vi "Example.vi"   [LabVIEW 2016, in "Global_logger.lvlib"]
uses:
  Global_logger.lvlib
  Levels.ctl
  Options.ctl
types:
  T1 = typedef "Global_logger.lvlib/Options.ctl" = cluster{"filesize (bytes)":u32, "logs max age (days) ":u16, "write per N messages":u16}
  T2 = typedef "Global_logger.lvlib/Levels.ctl" = enum16{"ALL", "TRACE", "DEBUG", "INFO", "WARN", "ERROR", "FATAL", "OFF"}
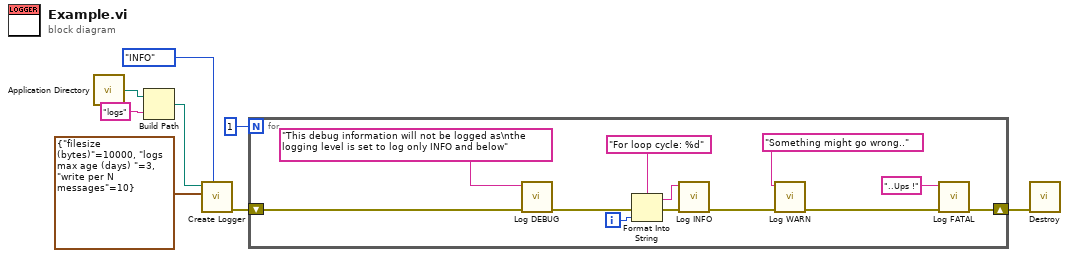
[diagram p0: block diagram]
diagram:
  n1 = call <vilib>:"Application Directory.vi"() -> ("Application Directory"=w6:path)
  n2 = Build Path(base path=w6, name or relative path="logs") -> (appended path=w4:path)
  n3 = call "Create Logger.vi"("Level"=Levels."INFO", "Options"=T1 {"filesize (bytes)"=10000, "logs max age (days) "=3, "write per N messages"=10}, "Root Logging Path"=w4) -> ("error out"=w3:errorcluster)  [unwired: 8 in]
  n4 = for {
    N: 1 -> [_]
    shift-right: [w17] -> w2
    shift-left: w3 -> [w20]
    i -> [w13]
    n5 = call "Log DEBUG.vi"("error in (no error)"=w20, "Message"="This debug information will not be logged as\nthe logging level is set to log only INFO and below") -> ("error out"=w19:errorcluster)  [unwired: 9 in]
    n6 = Format Into String(format string="For loop cycle: %d", error in=w19, w13) -> (resulting string=w11:string, error out=w14:errorcluster)  [unwired: 1 in]
    n7 = call "Log INFO.vi"("error in (no error)"=w14, "Message"=w11) -> ("error out"=w18:errorcluster)  [unwired: 9 in]
    n8 = call "Log WARN.vi"("error in (no error)"=w18, "Message"="Something might go wrong.." ("format string")) -> ("error out"=w10:errorcluster)  [unwired: 9 in]
    n9 = call "Log FATAL.vi"("error in (no error)"=w10, "Message"="..Ups !") -> ("error out"=w17:errorcluster)  [unwired: 9 in]
  }
  n10 = call "Destroy.vi"("error in (no error)"=w2) -> ()  [unwired: 10 in, 1 out]
